vi "Initialize.vi"(8 "error in (no error)":errorcluster, 11 "Ethernet in":refnum<class "TCP.lvclass">) -> (0 "error out":errorcluster, 3 "Ethernet out":refnum<class "TCP.lvclass">)   [LabVIEW 2019, in "Localhost Protocols.lvlib" / "TCP.lvclass"]
uses:
  TCP.lvclass
  TCP.lvclass/TCP.ctl
  Data Access/Read IP Address.vi
  Data Access/Read Port.vi
  Data Access/Write TCP Ref.vi
  Protocol Parent/Protocol Parent.lvclass
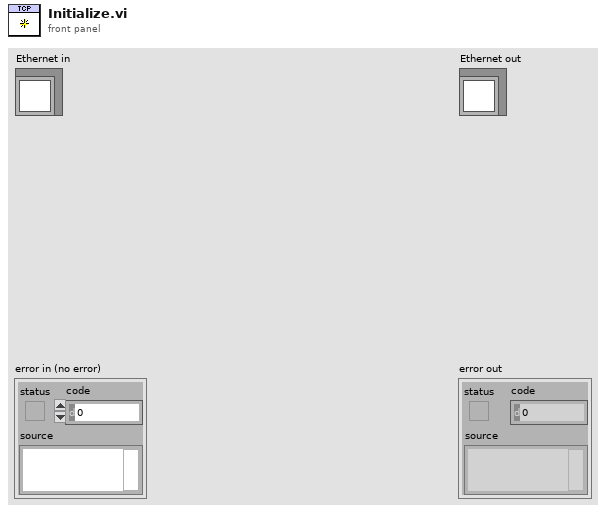
[diagram p1: front panel]
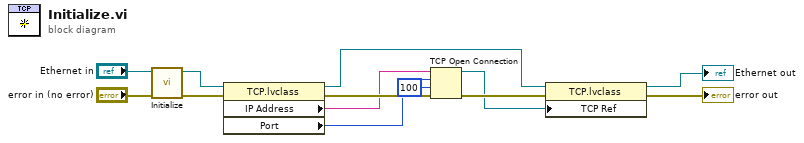
[diagram p0: block diagram]
diagram:
  n1 = call-parent "Initialize.vi"("error in (no error)"="error in (no error)", "Protocol Parent in"="Ethernet in") -> ("error out"=w11:errorcluster, "Protocol Parent out"=w10:refnum<class "TCP.lvclass">)  [unwired: 8 in]
  n2 = property class="TCP.lvclass"(reference=w10, error in=w11) -> (reference out=w4:refnum<class "TCP.lvclass">, error out=w9:errorcluster, "IP Address"=w8:string, "Port"=w7:u16)
  n3 = TCP Open Connection(address=w8, remote port or service name=w7, timeout ms (60000)=100, error in (no error)=w9) -> (connection ID=w2:refnum<k5>, error out=w6:errorcluster)  [unwired: 1 in]
  n4 = property class="TCP.lvclass"(reference=w4, error in=w6, "TCP Ref"=w2) -> (reference out=→"Ethernet out":refnum<class "TCP.lvclass">, error out=→"error out":errorcluster)
